vi "SVG Editing Playground.vi"() -> ()   [LabVIEW 2019]
uses:
  Classes/Parse/Image/SVGImage.lvclass
  Classes/Parse/ParseXML/ParseSVG.lvclass
  Classes/Parse/ParseXML/Image.ctl
  <vilib>/LabVIEW Open Source Project/Unicity/UniqueName/UniqueNameClass/Key.ctl
  <vilib>/LabVIEW Open Source Project/Unicity/UniqueName/UniquenessCriteria/Criteria.ctl
  Classes/Parse/ParseXML/ParseSVG.lvclass/ParseSVG.ctl
  <vilib>/LabVIEW Open Source Project/Unicity/UniqueName/UniqueNameClass/UniqueName.lvclass/UniqueName.ctl
  Classes/Parse/Image/InitializationInfo.ctl
  Classes/Parse/EditSVG/EditSVG.lvclass
  <vilib>/LabVIEW Open Source Project/Unicity/UniqueName/Registry/NameRegistry.lvclass
  <vilib>/LabVIEW Open Source Project/Unicity/UniqueName/UniqueNameClass/UniqueName.lvclass
  <vilib>/LabVIEW Open Source Project/Unicity/UniqueName/UniquenessCriteria/UniquenessCriteria.lvclass
panel:
  out "after substring":string
  out "offset past match 5":i32
  out "offset past match 4":i32
  out "offset past match 3":i32
  out "offset past match 2":i32
  out "Array 4":string[](array[string])
  out "Array 3":i32[](array[numeric])
  out "Array 2":i32[](array[numeric])
  out "Array":i32[](array[numeric])
  out "offset past match":i32
  out "Groups":T1(array[cluster])
  out "Path End":i32[](array[numeric])
  out "path start":i32[](array[numeric])
  in  "RawXML":string
  out "Edited in":string
  out "Background Image":refnum<class "SVGImage.lvclass">
  out "error out":errorcluster
  # "ff d8 ff e0 00 10 4a 46 49 46 00 01 01 00 00 01 00 01 00 00 ff fe 00 2d"
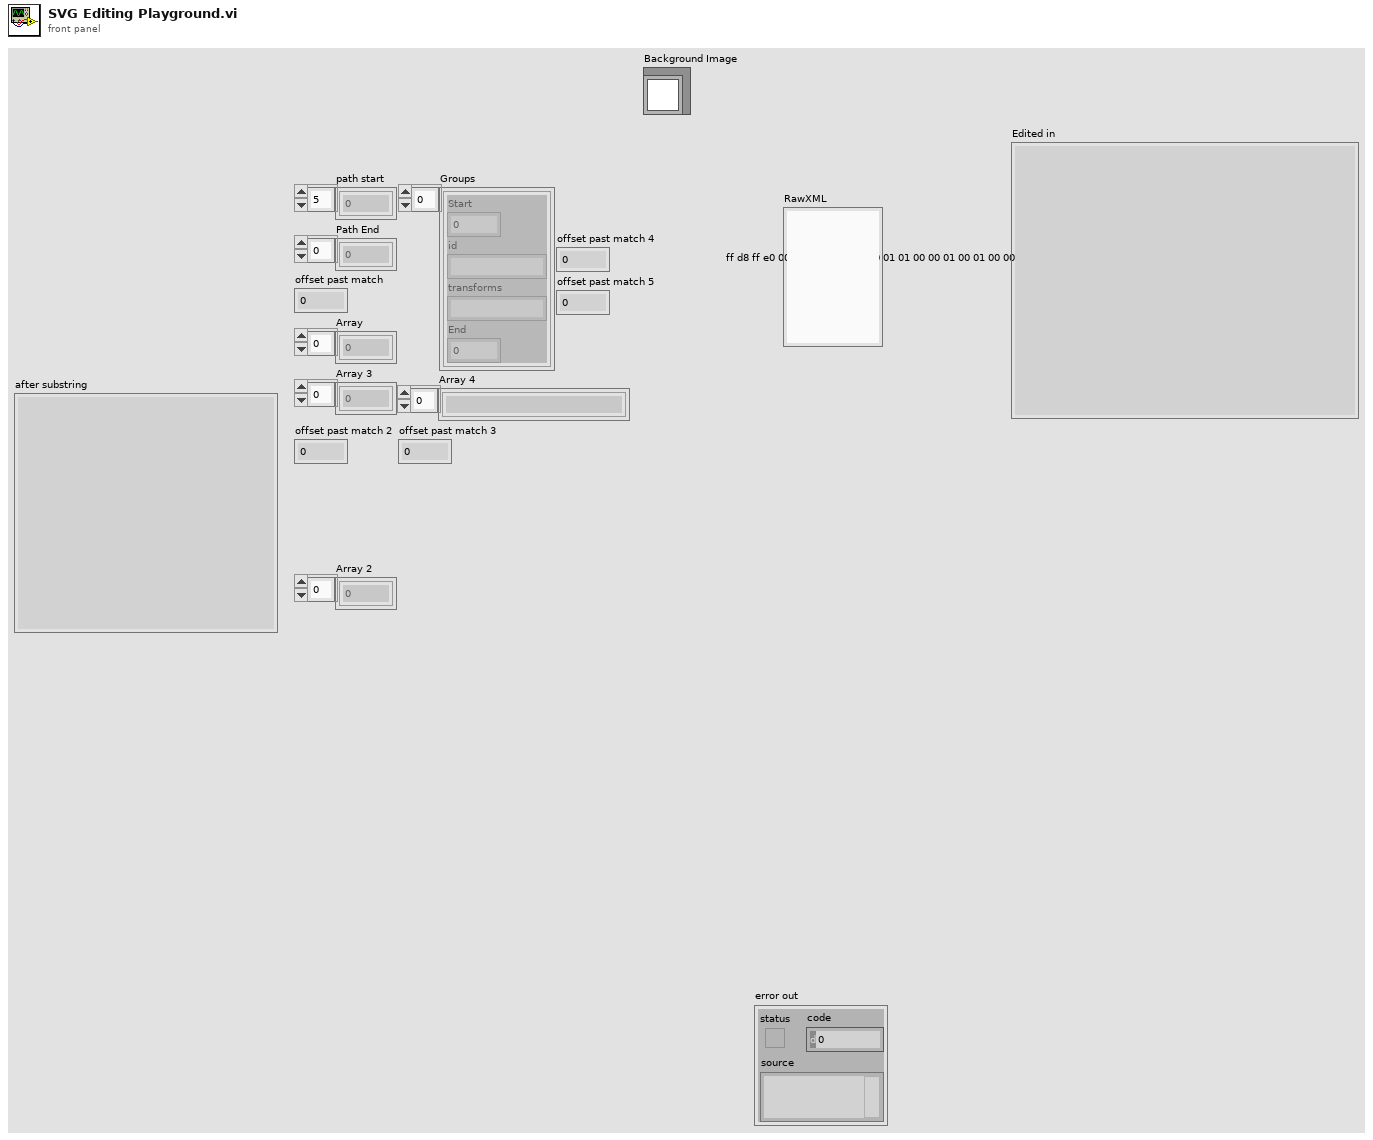
[diagram p1: front panel]
types:
  T1 = cluster{"Start":i32, "id":string, "transforms":string, "End":i32}[]
  T2 = typedef "UniqueName.lvlib/UniquenessCriteria.lvclass/Criteria.ctl" = enum16{"Globally-Unique Fully Qualified Name", "Globally-Unique Name", "Universal Unique Identifier"}
  T3 = typedef "UniqueName.lvlib/UniqueName.lvclass/Key.ctl" = enum16{"Fully Qualified Name", "Unique Name", "Given Name", "Parent Fully Qualified Name", "UUID"}
  T4 = cluster{"Start":i32, "attributes":string, "End":i32}
  T5 = typedef "ParseSVG.lvclass/Image.ctl" = cluster{"x":string, "y":string, "width":string, "height":string, "xlink:href":string, "id":string, "transform":string}
  T6 = typedef "UniqueName.lvlib/NameRegistry.lvclass/RegistryConfiguration.ctl" = cluster{"Delimiter":refnum<class "Delimiter.lvclass">, "RandomStringGenerator":refnum<class "RandomStringGenerator.lvclass">, "UniquenessCriteria":refnum<class "UniquenessCriteria.lvclass">, "StringIncrement":refnum<class "StringIncrement.lvclass">}
  T7 = typedef "SVGImage.lvclass/InitializationInfo.ctl" = cluster{"X":string, "Y":string, "Width":string, "Height":string, "File Path":string, "ID":string, "transform":string}
  T8 = cluster{"Backmost?":bool, "Correct location?":bool, "Surface Pic?":bool, "Correct Name?":bool}
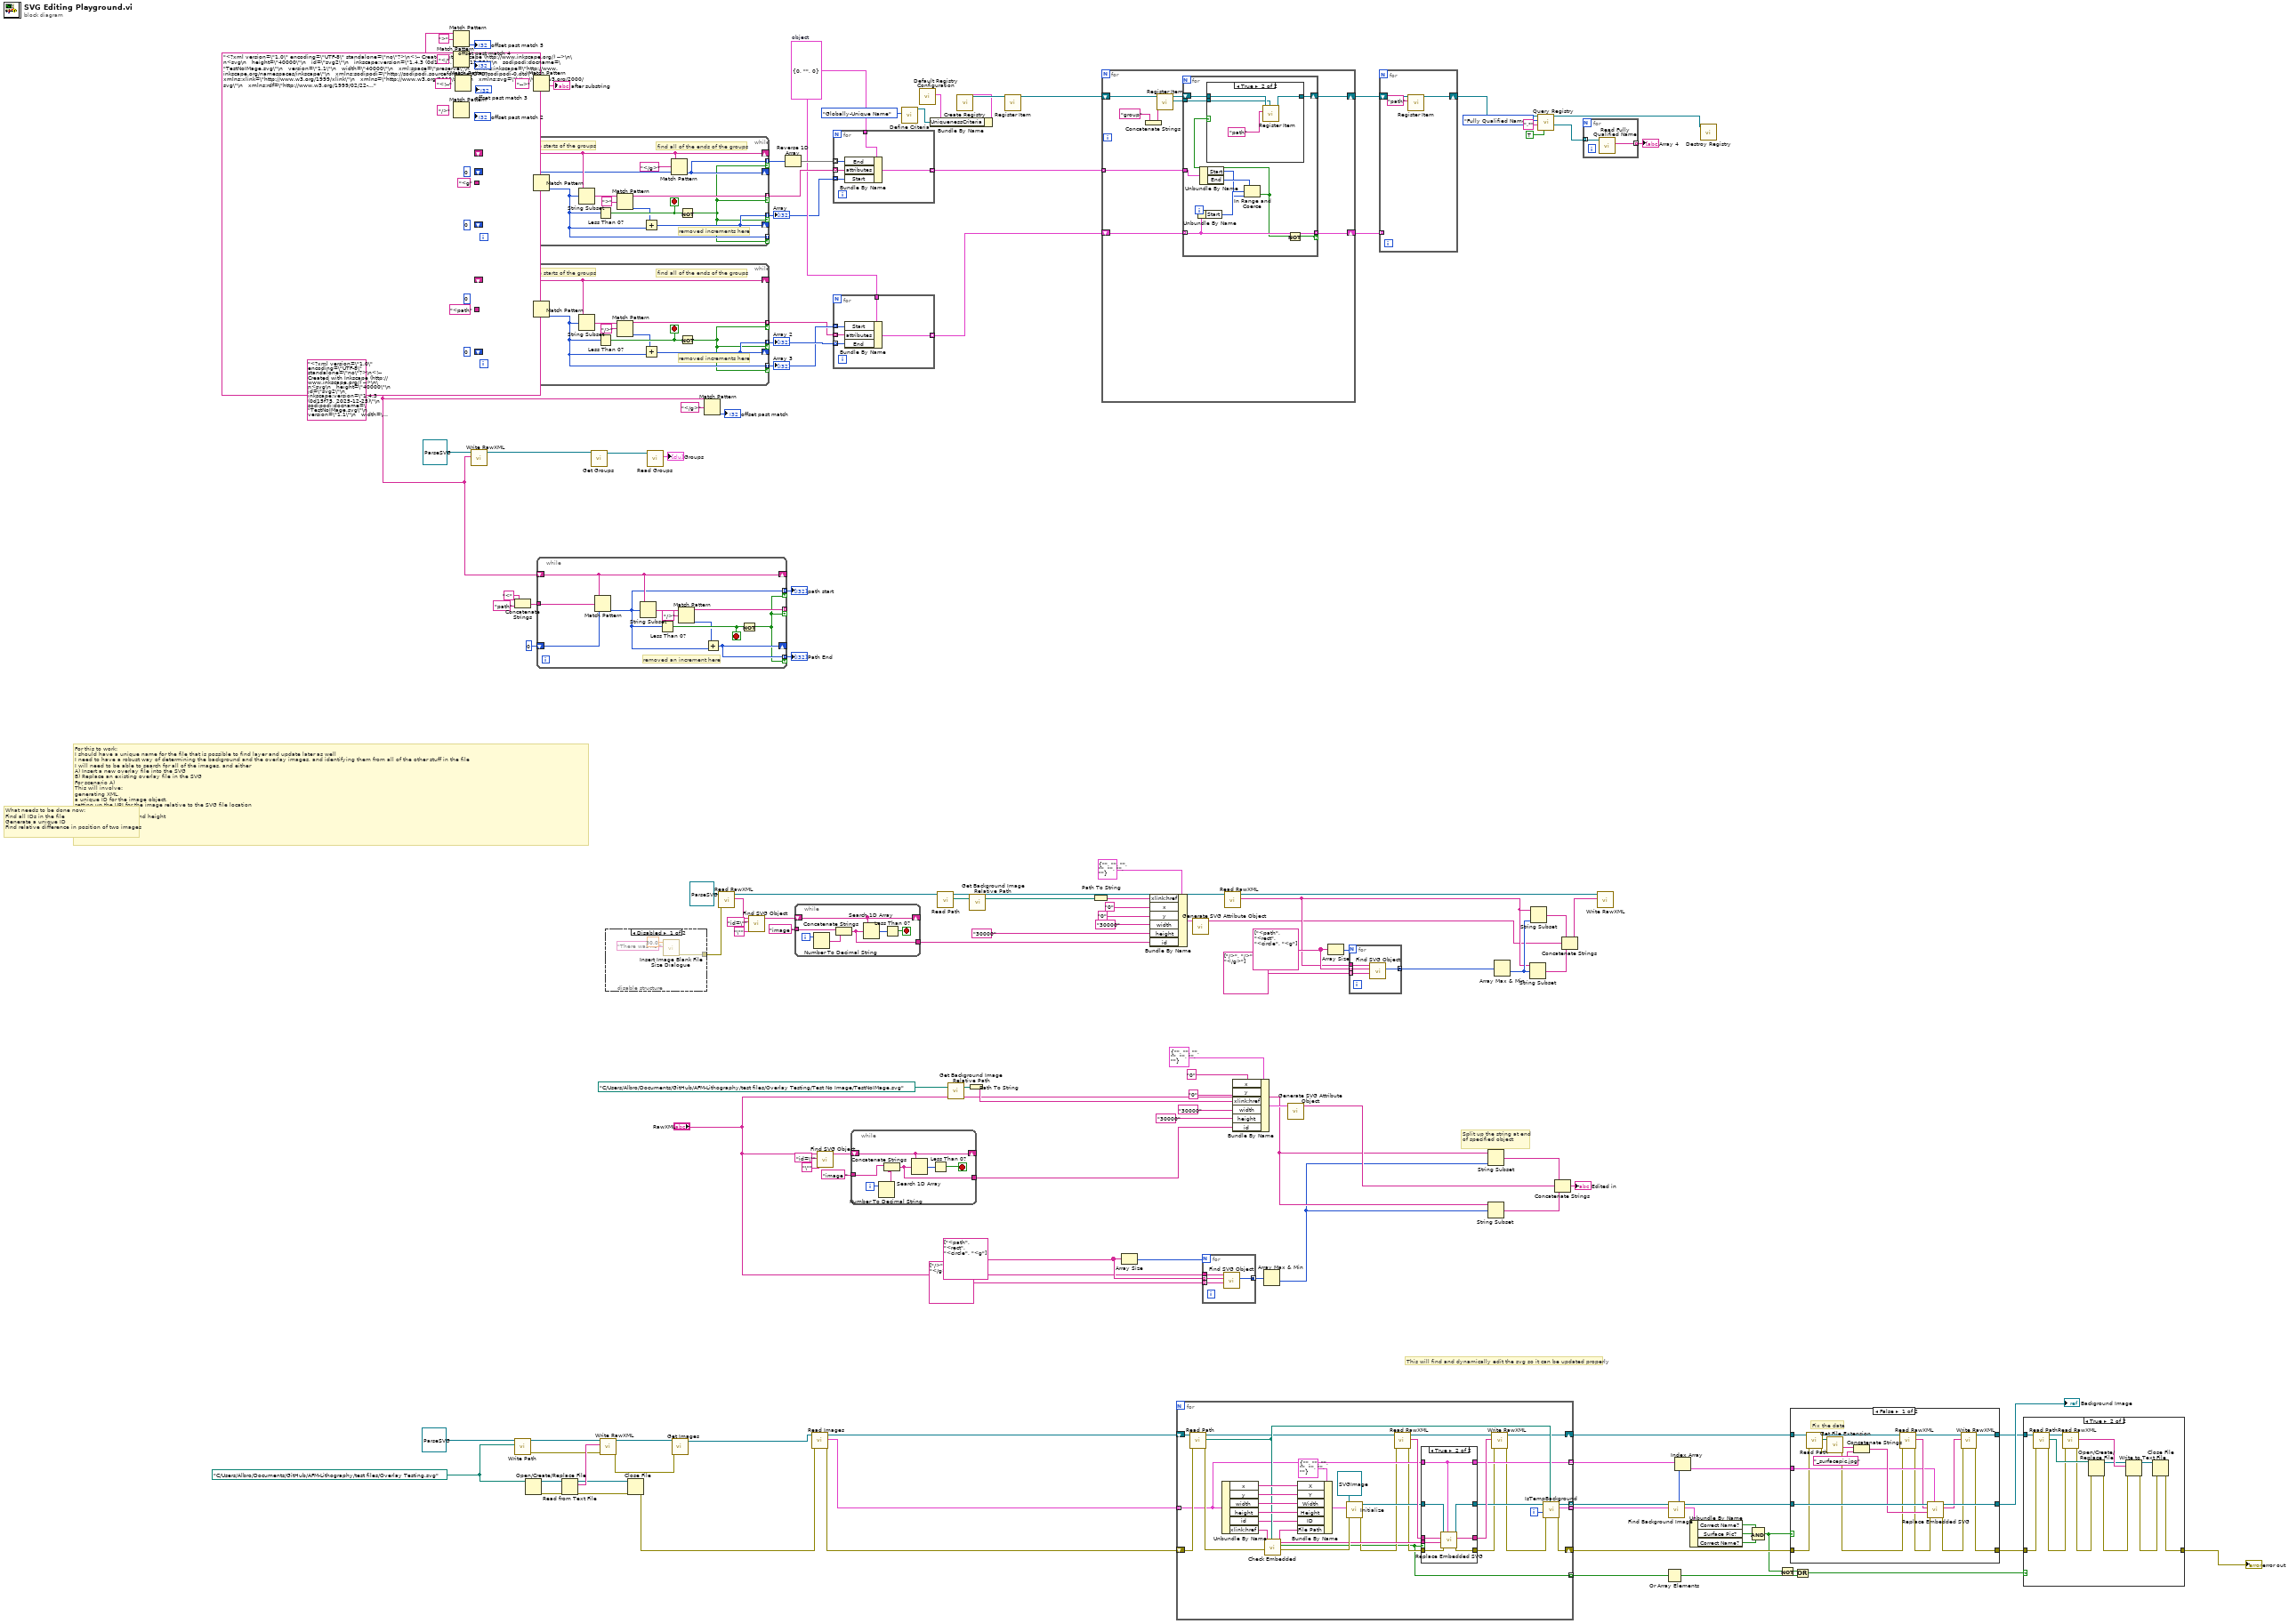
[diagram p0: block diagram]
diagram:
  w8 = "<?xml version=\"1.0\" encoding=\"UTF-8\" standalone=\"no\"?>\n<!-- Created with Inkscape (http://www.inkscape.org/) -->\n\n<svg\n   height=\"40000\"\n   id=\"svg2\"\n   inkscape:version=\"1.4.3 (0d15f75, 2025-12-25)\"\n   sodipodi:docname=\"TestNoIMage.svg\"\n   version=\"1.1\"\n   width=\"40000\"\n   xml:space=\"preserve\"\n   xmlns:inkscape=\"http://www.inkscape.org/namespaces/inkscape\"\n   xmlns:sodipodi=\"http://sodipodi.sourceforge.net/DTD/sodipodi-0.dtd\"\n   xmlns:xlink=\"http://www.w3.org/1999/xlink\"\n   xmlns=\"http://www.w3.org/2000/svg\"\n   xmlns:svg=\"http://www.w3.org/2000/svg\"\n   xmlns:rdf=\"http://www.w3.org/1999/02/22-rdf-syntax-ns#\"\n   xmlns:cc=\"http://creativecommons.org/ns#\"\n   xmlns:dc=\"http://purl.org/dc/elements/1.1/\"><sodipodi:namedview\n     bordercolor=\"#666666\"\n     borderopacity=\"1.0\"\n     id=\"base\"\n     inkscape:current-layer=\"svg2\"\n     inkscape:cx=\"5250\"\n     inkscape:cy=\"13700\"\n     inkscape:deskcolor=\"#d1d1d1\"\n     inkscape:document-units=\"px\"\n     inkscape:pagecheckerboard=\"0\"\n     inkscape:pageopacity=\"0.0\"\n     inkscape:pageshadow=\"2\"\n     inkscape:showpageshadow=\"false\"\n     inkscape:window-height=\"991\"\n     inkscape:window-maximized=\"1\"\n     inkscape:window-width=\"1920\"\n     inkscape:window-x=\"-9\"\n     inkscape:window-y=\"-9\"\n     inkscape:zoom=\"0.01\"\n     pagecolor=\"#ffffff\"\n     showgrid=\"false\" /><defs\n     id=\"defs4\" /><metadata\n     id=\"metadata7\"><rdf:RDF><cc:Work\n         rdf:about=\"\"><dc:format>image/svg+xml</dc:format><dc:type\n           rdf:resource=\"http://purl.org/dc/dcmitype/StillImage\" /></cc:Work></rdf:RDF></metadata><image\n     x=\"0\"\n     y=\"0\"\n     width=\"40000\"\n     height=\"40000\"\n     xlink:href=\"TestNoIMage_surfacepic.jpg\"\n     id=\"image 0\" /><path\n     d=\"m 5710.9429,17975.706 44.593,-4593.756 c 1461.0246,971.983 3035.6976,1713.83 4682.3101,2310.003 -1752.8115,344.069 -3431.5235,862.613 -4726.9031,2283.753 z\"\n     id=\"path3768\"\n     inkscape:connector-curvature=\"0\"\n     sodipodi:nodetypes=\"cccc\"\n     style=\"fill:#00ff00;fill-opacity:1;stroke:#00fb00;stroke-width:68.42746735;stroke-linecap:butt;stroke-linejoin:miter;stroke-miterlimit:4;stroke-dasharray:none;stroke-opacity:1\" /><path\n     d=\"m 13400.892,10059.383 4593.756,44.594 c -971.983,1461.024 -1713.83,3035.698 -2310.003,4682.311 -344.069,-1752.812 -862.613,-3431.524 -2283.753,-4726.905 z\"\n     id=\"path3768-1\"\n     inkscape:connector-curvature=\"0\"\n     sodipodi:nodetypes=\"cccc\"\n     style=\"fill:#00ff00;fill-opacity:1;stroke:#00fb00;stroke-width:68.42746735;stroke-linecap:butt;stroke-linejoin:miter;stroke-miterlimit:4;stroke-dasharray:none;stroke-opacity:1\" /><path\n     d=\"m 18739.549,9988.6728 4593.756,44.5932 c -971.983,1461.025 -1713.83,3035.698 -2310.003,4682.311 -344.069,-1752.812 -862.613,-3431.524 -2283.753,-4726.9042 z\"\n     id=\"path3768-9\"\n     inkscape:connector-curvature=\"0\"\n     sodipodi:nodetypes=\"cccc\"\n     style=\"fill:#00ff00;fill-opacity:1;stroke:#00fb00;stroke-width:68.42746735;stroke-linecap:butt;stroke-linejoin:miter;stroke-miterlimit:4;stroke-dasharray:none;stroke-opacity:1\" /><path\n     d=\"m 8100.4383,10879.12 4509.0037,-879.4745 c -658.548,1626.5485 -1068.815,3318.1785 -1321.924,5051.0065 -689.294,-1647.91 -1534.6121,-3188.17 -3187.0797,-4171.532 z\"\n     id=\"path3768-88\"\n     inkscape:connector-curvature=\"0\"\n     sodipodi:nodetypes=\"cccc\"\n     style=\"fill:#00ff00;fill-opacity:1;stroke:#00fb00;stroke-width:68.42746735;stroke-linecap:butt;stroke-linejoin:miter;stroke-miterlimit:4;stroke-dasharray:none;stroke-opacity:1\" /><path\n     d=\"M 28994.557,10486.846 25071.601,9220.3251 c 541.997,1669.0069 177.663,3332.3599 307.727,5078.7399 803.986,-1595.099 1897.423,-2948.05 3615.229,-3812.219 z\"\n     id=\"path3768-88-4\"\n     inkscape:connector-curvature=\"0\"\n     sodipodi:nodetypes=\"cccc\"\n     style=\"fill:#00ff00;fill-opacity:1;stroke:#00fb00;stroke-width:68.4275;stroke-linecap:butt;stroke-linejoin:miter;stroke-miterlimit:4;stroke-dasharray:none;stroke-opacity:1\" /><path\n     d=\"m 31708.383,17654.207 -44.593,-4593.756 c -1461.024,971.983 -3035.697,1713.83 -4682.31,2310.003 1752.812,344.069 3431.524,862.613 4726.903,2283.753 z\"\n     id=\"path3768-3\"\n     inkscape:connector-curvature=\"0\"\n     sodipodi:nodetypes=\"cccc\"\n     style=\"fill:#00ff00;fill-opacity:1;stroke:#00fb00;stroke-width:68.42746735;stroke-linecap:butt;stroke-linejoin:miter;stroke-miterlimit:4;stroke-dasharray:none;stroke-opacity:1\" /><path\n     d=\"m 9075.4469,21348.552 c 0,0 -5.0869,-1278.12 199.2302,-1901.329 280.3951,-855.263 106.6737,-1996.952 1394.6099,-2478.519 1377.731,-515.142 5080.057,-279.059 7627.666,-339.523 1876.994,-44.548 3759.094,-71.272 5635.365,-16.976 1209.741,35.007 2679.222,-238.229 3614.603,220.69 903.916,443.482 984.374,1305.486 1024.612,2003.186 44.859,777.835 -882.304,2274.805 -882.304,2274.805\"\n     id=\"path3856\"\n     inkscape:connector-curvature=\"0\"\n     sodipodi:nodetypes=\"casaaaac\"\n     style=\"fill:none;stroke:#00fb00;stroke-width:62.17174911;stroke-linecap:butt;stroke-linejoin:miter;stroke-miterlimit:4;stroke-dasharray:none;stroke-opacity:1\" /><rect\n     height=\"7255.8125\"\n     id=\"rect14\"\n     style=\"opacity:1;fill:#00ff00;fill-opacity:1;stroke:#000000;stroke-width:0.755906;stroke-miterlimit:4;stroke-dasharray:none;stroke-opacity:1\"\n     width=\"11888.403\"\n     x=\"14347.161\"\n     y=\"20973.98\" /><rect\n     height=\"7253.042\"\n     id=\"rect14-8\"\n     style=\"fill:#00ff00;fill-opacity:1;stroke:#000000;stroke-width:0.693561;stroke-miterlimit:4;stroke-dasharray:none;stroke-opacity:1\"\n     transform=\"matrix(1.1237265,-0.00330692,0.45761161,1.2541239,-10097.789,-20728.359)\"\n     width=\"10291.699\"\n     x=\"-4974.5957\"\n     y=\"39154.031\" /><text\n     id=\"text843\"\n     style=\"font-style:normal;font-weight:normal;font-size:53.3333px;line-height:1.25;font-family:sans-serif;letter-spacing:0px;word-spacing:0px;fill:#000000;fill-opacity:1;stroke:none\"\n     x=\"12020.815\"\n     xml:space=\"preserve\"\n     y=\"20554.562\">\n    <tspan\n   id=\"tspan841\"\n   sodipodi:role=\"line\"\n   x=\"12020.815\"\n   y=\"20554.562\">T</tspan>\n  </text><circle\n     cx=\"15000\"\n     cy=\"18500\"\n     id=\"path825\"\n     r=\"100\"\n     style=\"opacity:1;fill:#00ff00;fill-opacity:1;stroke:#000000;stroke-width:1.00157;stroke-miterlimit:4;stroke-dasharray:none;stroke-opacity:1\" /><circle\n     cx=\"20000\"\n     cy=\"18500\"\n     id=\"path825-31\"\n     r=\"100\"\n     style=\"fill:#00ff00;fill-opacity:1;stroke:#000000;stroke-width:1.00157;stroke-miterlimit:4;stroke-dasharray:none;stroke-opacity:1\" /><circle\n     cx=\"22500\"\n     cy=\"18500\"\n     id=\"path825-3\"\n     r=\"100\"\n     style=\"fill:#00ff00;fill-opacity:1;stroke:#000000;stroke-width:1.00157;stroke-miterlimit:4;stroke-dasharray:none;stroke-opacity:1\" /><circle\n     cx=\"17500\"\n     cy=\"18500\"\n     id=\"path825-9\"\n     r=\"100\"\n     style=\"fill:#00ff00;fill-opacity:1;stroke:#000000;stroke-width:1.00157;stroke-miterlimit:4;stroke-dasharray:none;stroke-opacity:1\" /><circle\n     cx=\"25000\"\n     cy=\"18500\"\n     id=\"path825-3-5\"\n     r=\"100\"\n     style=\"fill:#00ff00;fill-opacity:1;stroke:#000000;stroke-width:1.00157;stroke-miterlimit:4;stroke-dasharray:none;stroke-opacity:1\" /><circle\n     cx=\"13000\"\n     cy=\"20500\"\n     id=\"path825-5\"\n     r=\"100\"\n     style=\"fill:#00ff00;fill-opacity:1;stroke:#000000;stroke-width:1.00157;stroke-miterlimit:4;stroke-dasharray:none;stroke-opacity:1\" /><circle\n     cx=\"17000\"\n     cy=\"20500\"\n     id=\"path825-3-4\"\n     r=\"100\"\n     style=\"fill:#00ff00;fill-opacity:1;stroke:#000000;stroke-width:1.00157;stroke-miterlimit:4;stroke-dasharray:none;stroke-opacity:1\" /><circle\n     cx=\"15000\"\n     cy=\"20500\"\n     id=\"path825-9-6\"\n     r=\"100\"\n     style=\"fill:#00ff00;fill-opacity:1;stroke:#000000;stroke-width:1.00157;stroke-miterlimit:4;stroke-dasharray:none;stroke-opacity:1\" /><circle\n     cx=\"19000\"\n     cy=\"20500\"\n     id=\"path825-3-5-2\"\n     r=\"100\"\n     style=\"fill:#00ff00;fill-opacity:1;stroke:#000000;stroke-width:1.00157;stroke-miterlimit:4;stroke-dasharray:none;stroke-opacity:1\" /><path\n     d=\"M 13650,17000 26000,15600\"\n     id=\"path1392\"\n     inkscape:connector-curvature=\"0\"\n     style=\"fill:none;stroke:#00ff00;stroke-width:50;stroke-linecap:butt;stroke-linejoin:miter;stroke-miterlimit:4;stroke-dasharray:none;stroke-opacity:1\" /><path\n     d=\"m 11200,26850 c 1203.007,3334.458 2168.666,2633.989 3250,3900 l 3300,-1750\"\n     id=\"path1394\"\n     inkscape:connector-curvature=\"0\"\n     sodipodi:nodetypes=\"ccc\"\n     style=\"fill:none;stroke:#00ff00;stroke-width:50;stroke-linecap:butt;stroke-linejoin:miter;stroke-miterlimit:4;stroke-dasharray:none;stroke-opacity:1\" /><path\n     d=\"m 14849.242,3959.7979 h 11525.84\"\n     id=\"path4\"\n     style=\"fill:none;stroke:#00ff00;stroke-width:100px;stroke-linecap:butt;stroke-linejoin:miter;stroke-opacity:1\"\n     transform=\"translate(0,440)\" /><path\n     d=\"M 14849.242,4560.8386 H 26357.405\"\n     id=\"path2\"\n     style=\"fill:none;stroke:#00FF00;stroke-width:100px;stroke-linecap:butt;stroke-linejoin:miter;stroke-opacity:1\" /><g\n     id=\"g1\"\n     transform=\"matrix(0.97420092,0,0,1.1904169,383.55282,-892.60137)\"><path\n       d=\"M 14850,5174.9999 H 26349.999\"\n       id=\"path1\"\n       style=\"fill:none;stroke:#00ff00;stroke-width:100px;stroke-linecap:butt;stroke-linejoin:miter;stroke-opacity:1\"\n       transform=\"translate(16.91967,-437.3846)\" /><g\n       id=\"g3\"\n       transform=\"matrix(0.87240932,-0.1215228,0.11425413,0.92791062,3276.3322,3478.6107)\"><path\n         d=\"m 14849.242,3959.7979 h 11525.84\"\n         id=\"path4-6\"\n         style=\"fill:none;stroke:#00ff00;stroke-width:100px;stroke-linecap:butt;stroke-linejoin:miter;stroke-opacity:1\"\n         transform=\"translate(4993.758,1820.2021)\" /><path\n         d=\"M 14849.242,4560.8386 H 26357.405\"\n         id=\"path2-3\"\n         style=\"fill:none;stroke:#00ff00;stroke-width:100px;stroke-linecap:butt;stroke-linejoin:miter;stroke-opacity:1\"\n         transform=\"translate(4993.758,1380.2021)\" /><path\n         d=\"M 14850,5174.9999 H 26349.999\"\n         id=\"path1-6\"\n         style=\"fill:none;stroke:#00ff00;stroke-width:100px;stroke-linecap:butt;stroke-linejoin:miter;stroke-opacity:1\"\n         transform=\"translate(5010.6777,942.8175)\" /></g></g><path\n     d=\"M 19657.6 32703.7 C 19692.2 32408.2 19726.9 32124.8 19761.6 32036.9 C 19796.2 31949 19830.9 32064.5 19865.6 32307.7 C 19900.2 32551 19934.9 32903 19969.6 33135.3 C 20004.2 33367.7 20038.9 33461.2 20073.6 33356 C 20108.2 33250.7 20142.9 32954.3 20177.6 32659.4 C 20212.2 32364.5 20246.9 32094.9 20281.6 32025.1 C 20316.2 31955.3 20350.9 32091.6 20385.6 32345 C 20420.2 32598.4 20454.9 32949 20489.6 33169.3 C 20524.3 33389.6 20558.9 33461.4 20593.6 33338.9 C 20628.3 33216.3 20662.9 32908.4 20697.6 32615.3 C 20732.3 32322.2 20766.9 32067.5 20801.6 32016 C 20836.3 31964.5 20870.9 32121.2 20905.6 32383.7 C 20940.3 32646.2 20974.9 32994 21009.6 33201.3 C 21044.3 33408.7 21078.9 33458.5 21113.6 33319.2 C 21148.3 33179.8 21182.9 32861.7 21217.6 32571.5 C 21252.3 32281.4 21286.9 32042.7 21321.6 32009.7 C 21356.3 31976.8 21390.9 32153.1 21425.6 32423.7 C 21460.3 32694.3 21494.9 33037.8 21529.6 33231.4 C 21564.3 33425 21598.9 33452.6 21633.6 33297 C 21668.3 33141.4 21702.9 32814.3 21737.6 32528.3 C 21772.3 32242.3 21806.9 32020.5 21841.6 32006.2 C 21876.3 31992 21910.9 32187.3 21945.6 32464.9 C 21980.3 32742.4 22014.9 33080.3 22049.6 33259.3 C 22084.3 33438.4 22119 33443.7 22153.6 33272.5 C 22188.3 33101.3 22223 32766.6 22257.6 32485.8 C 22292.3 32205.1 22327 32001 22361.6 32005.5 C 22396.3 32010 22431 32223.5 22465.6 32507 C 22500.3 32790.4 22535 33121.2 22569.6 33285 C 22604.3 33448.9 22639 33431.8 22673.6 33245.6 C 22708.3 33059.5 22743 32718.5 22777.6 32444.2 C 22812.3 32169.8 22847 31984.4 22881.6 32007.6 C 22916.3 32030.8 22951 32261.7 22985.6 32549.9 C 23020.3 32838 23055 33160.5 23089.6 33308.4 C 23124.3 33456.3 23159 33417 23193.6 33216.6 C 23228.3 33016.3 23263 32670.4 23297.6 32403.6 C 23332.3 32136.7 23367 31970.7 23401.6 32012.5 C 23436.3 32054.4 23471 32301.7 23505.6 32593.4 C 23540.3 32885.1 23575 33198 23609.6 33329.3 C 23644.3 33460.7 23679 33399.2 23713.6 33185.5 C 23748.3 32971.9 23783 32622.5 23817.7 32364.2 C 23852.3 32105.9 23887 31959.9 23921.7 32020.2 C 23956.3 32080.5 23991 32343.2 24025.7 32637.3 C 24060.3 32931.4 24095 33233.4 24129.7 33347.7 C 24164.3 33462.1 24199 33378.7 24233.7 33152.5 C 24268.3 32926.3 24303 32574.8 24337.7 32326.2 C 24372.3 32077.5 24407 31952.1 24441.7 32030.7 C 24476.3 32109.2 24511 32386.2 24545.7 32681.5 C 24580.3 32976.8 24615 33266.7 24649.7 33363.6 C 24684.3 33460.4 24719 33355.5 24753.7 33117.7 C 24788.3 32879.9 24823 32527.7 24857.7 32289.7 C 24892.3 32051.7 24927 31947.4 24961.7 32043.8 C 24996.3 32140.3 25031 32430.5 25065.7 32725.8 C 25100.3 33021.1 25135 33297.8 25169.7 33376.7 C 25204.3 33455.6 25239 33329.6 25273.7 33081.2 C 25308.3 32832.8 25343 32481.3 25377.7 32254.9 C 25412.3 32028.4 25447 31945.7 25481.7 32059.6 C 25516.4 32173.6 25551 32475.9 25585.7 32770.1 C 25620.4 33064.2 25655 33326.5 25689.7 33387.2 C 25724.4 33447.8 25759 33301.3 25793.7 33043.2 C 25828.4 32785.1 25863 32435.8 25897.7 32221.8 C 25932.4 32007.9 25967 31947 26001.7 32078 C 26036.4 32209.1 26071 32522.3 26105.7 32814 C 26140.4 33105.8 26175 33352.6 26209.7 33394.8 C 26244.4 33437.1 26279 33270.5 26313.7 33003.8 C 26348.4 32737.1 26383 32391.3 26417.7 32190.7 C 26452.4 31990.1 26487 31951.4 26521.7 32099 C 26556.4 32246.5 26591 32569.3 26625.7 32857.5 C 26660.4 33145.8 26695 33376.2 26729.7 33399.8 C 26764.4 33423.4 26799 33237.4 26833.7 32963.2 C 26868.4 32689 26903 32348.2 26937.7 32161.7 C 26972.4 31975.3 27007 31958.8 27041.7 32122.3 C 27076.4 32285.8 27111 32616.9 27145.7 32900.4 C 27180.4 33183.9 27215.1 33397 27249.7 33401.9 C 27284.4 33406.7 27319.1 33202.2 27353.7 32921.6 C 27388.4 32640.9 27423.1 32306.4 27457.7 32134.9 C 27492.4 31963.4 27527.1 31969.3 27561.7 32148 C 27596.4 32326.8 27631.1 32664.8 27665.7 32942.5 C 27700.4 33220.2 27735.1 33415 27769.7 33401.2 C 27804.4 33387.3 27839.1 33165 27873.7 32879.1 C 27908.4 32593.1 27943.1 32266.3 27977.7 32110.4 C 28012.4 31954.4 28047.1 31982.6 28081.7 32176 C 28116.4 32369.3 28151.1 32712.9 28185.7 32983.6 C 28220.4 33254.4 28255.1 33430.2 28289.7 33397.7 C 28324.4 33365.1 28359.1 33125.9 28393.7 32835.8 C 28428.4 32545.8 28463.1 32227.9 28497.7 32088.2 C 28532.4 31948.5 28567.1 31998.9 28601.7 32206 C 28636.4 32413.2 28671.1 32761 28705.7 33023.7 C 28740.4 33286.3 28775.1 33442.5 28809.8 33391.3 C 28844.4 33340.2 28879.1 33085.1 28913.8 32792.1 C 28948.4 32499 28983.1 32191.4 29017.8 32068.5 C 29052.4 31945.6 29087.1 32018 29121.8 32238.1 C 29156.4 32458.2 29191.1 32808.8 29225.8 33062.4 C 29260.4 33316 29295.1 33451.7 29329.8 33382.3 C 29364.4 33312.8 29399.1 33042.8 29433.8 32748 C 29468.4 32453.1 29503.1 32157 29537.8 32051.4 C 29572.4 31945.8 29607.1 32039.9 29641.8 32272 C 29676.4 32504.2 29711.1 32856.2 29745.8 33099.6 C 29780.4 33343.1 29815.1 33458 29849.8 33370.5 C 29884.4 33282.9 29919.1 32999.1 29953.8 32703.7\"\n     id=\"path3\"\n     style=\"fill:none;stroke:#00ff00;stroke-width:100;paint-order:fill markers stroke;stroke-dasharray:none\"\n     title=\"t sin(20*t)\" /></svg>"
  (unwired) 0 ("offset past match")
  w34 = T4 {"Start"=0, "attributes"="", "End"=0}  # object
  w37 = "<?xml version=\"1.0\" encoding=\"UTF-8\" standalone=\"no\"?>\n<!-- Created with Inkscape (http://www.inkscape.org/) -->\n\n<svg\n   height=\"40000\"\n   id=\"svg2\"\n   inkscape:version=\"1.4.3 (0d15f75, 2025-12-25)\"\n   sodipodi:docname=\"TestNoIMage.svg\"\n   version=\"1.1\"\n   width=\"40000\"\n   xml:space=\"preserve\"\n   xmlns:inkscape=\"http://www.inkscape.org/namespaces/inkscape\"\n   xmlns:sodipodi=\"http://sodipodi.sourceforge.net/DTD/sodipodi-0.dtd\"\n   xmlns:xlink=\"http://www.w3.org/1999/xlink\"\n   xmlns=\"http://www.w3.org/2000/svg\"\n   xmlns:svg=\"http://www.w3.org/2000/svg\"\n   xmlns:rdf=\"http://www.w3.org/1999/02/22-rdf-syntax-ns#\"\n   xmlns:cc=\"http://creativecommons.org/ns#\"\n   xmlns:dc=\"http://purl.org/dc/elements/1.1/\"><sodipodi:namedview\n     bordercolor=\"#666666\"\n     borderopacity=\"1.0\"\n     id=\"base\"\n     inkscape:current-layer=\"svg2\"\n     inkscape:cx=\"5250\"\n     inkscape:cy=\"13700\"\n     inkscape:deskcolor=\"#d1d1d1\"\n     inkscape:document-units=\"px\"\n     inkscape:pagecheckerboard=\"0\"\n     inkscape:pageopacity=\"0.0\"\n     inkscape:pageshadow=\"2\"\n     inkscape:showpageshadow=\"false\"\n     inkscape:window-height=\"991\"\n     inkscape:window-maximized=\"1\"\n     inkscape:window-width=\"1920\"\n     inkscape:window-x=\"-9\"\n     inkscape:window-y=\"-9\"\n     inkscape:zoom=\"0.01\"\n     pagecolor=\"#ffffff\"\n     showgrid=\"false\" /><defs\n     id=\"defs4\" /><metadata\n     id=\"metadata7\"><rdf:RDF><cc:Work\n         rdf:about=\"\"><dc:format>image/svg+xml</dc:format><dc:type\n           rdf:resource=\"http://purl.org/dc/dcmitype/StillImage\" /></cc:Work></rdf:RDF></metadata><image\n     x=\"0\"\n     y=\"0\"\n     width=\"40000\"\n     height=\"40000\"\n     xlink:href=\"TestNoIMage_surfacepic.jpg\"\n     id=\"image 0\" /><path\n     d=\"m 5710.9429,17975.706 44.593,-4593.756 c 1461.0246,971.983 3035.6976,1713.83 4682.3101,2310.003 -1752.8115,344.069 -3431.5235,862.613 -4726.9031,2283.753 z\"\n     id=\"path3768\"\n     inkscape:connector-curvature=\"0\"\n     sodipodi:nodetypes=\"cccc\"\n     style=\"fill:#00ff00;fill-opacity:1;stroke:#00fb00;stroke-width:68.42746735;stroke-linecap:butt;stroke-linejoin:miter;stroke-miterlimit:4;stroke-dasharray:none;stroke-opacity:1\" /><path\n     d=\"m 13400.892,10059.383 4593.756,44.594 c -971.983,1461.024 -1713.83,3035.698 -2310.003,4682.311 -344.069,-1752.812 -862.613,-3431.524 -2283.753,-4726.905 z\"\n     id=\"path3768-1\"\n     inkscape:connector-curvature=\"0\"\n     sodipodi:nodetypes=\"cccc\"\n     style=\"fill:#00ff00;fill-opacity:1;stroke:#00fb00;stroke-width:68.42746735;stroke-linecap:butt;stroke-linejoin:miter;stroke-miterlimit:4;stroke-dasharray:none;stroke-opacity:1\" /><path\n     d=\"m 18739.549,9988.6728 4593.756,44.5932 c -971.983,1461.025 -1713.83,3035.698 -2310.003,4682.311 -344.069,-1752.812 -862.613,-3431.524 -2283.753,-4726.9042 z\"\n     id=\"path3768-9\"\n     inkscape:connector-curvature=\"0\"\n     sodipodi:nodetypes=\"cccc\"\n     style=\"fill:#00ff00;fill-opacity:1;stroke:#00fb00;stroke-width:68.42746735;stroke-linecap:butt;stroke-linejoin:miter;stroke-miterlimit:4;stroke-dasharray:none;stroke-opacity:1\" /><path\n     d=\"m 8100.4383,10879.12 4509.0037,-879.4745 c -658.548,1626.5485 -1068.815,3318.1785 -1321.924,5051.0065 -689.294,-1647.91 -1534.6121,-3188.17 -3187.0797,-4171.532 z\"\n     id=\"path3768-88\"\n     inkscape:connector-curvature=\"0\"\n     sodipodi:nodetypes=\"cccc\"\n     style=\"fill:#00ff00;fill-opacity:1;stroke:#00fb00;stroke-width:68.42746735;stroke-linecap:butt;stroke-linejoin:miter;stroke-miterlimit:4;stroke-dasharray:none;stroke-opacity:1\" /><path\n     d=\"M 28994.557,10486.846 25071.601,9220.3251 c 541.997,1669.0069 177.663,3332.3599 307.727,5078.7399 803.986,-1595.099 1897.423,-2948.05 3615.229,-3812.219 z\"\n     id=\"path3768-88-4\"\n     inkscape:connector-curvature=\"0\"\n     sodipodi:nodetypes=\"cccc\"\n     style=\"fill:#00ff00;fill-opacity:1;stroke:#00fb00;stroke-width:68.4275;stroke-linecap:butt;stroke-linejoin:miter;stroke-miterlimit:4;stroke-dasharray:none;stroke-opacity:1\" /><path\n     d=\"m 31708.383,17654.207 -44.593,-4593.756 c -1461.024,971.983 -3035.697,1713.83 -4682.31,2310.003 1752.812,344.069 3431.524,862.613 4726.903,2283.753 z\"\n     id=\"path3768-3\"\n     inkscape:connector-curvature=\"0\"\n     sodipodi:nodetypes=\"cccc\"\n     style=\"fill:#00ff00;fill-opacity:1;stroke:#00fb00;stroke-width:68.42746735;stroke-linecap:butt;stroke-linejoin:miter;stroke-miterlimit:4;stroke-dasharray:none;stroke-opacity:1\" /><path\n     d=\"m 9075.4469,21348.552 c 0,0 -5.0869,-1278.12 199.2302,-1901.329 280.3951,-855.263 106.6737,-1996.952 1394.6099,-2478.519 1377.731,-515.142 5080.057,-279.059 7627.666,-339.523 1876.994,-44.548 3759.094,-71.272 5635.365,-16.976 1209.741,35.007 2679.222,-238.229 3614.603,220.69 903.916,443.482 984.374,1305.486 1024.612,2003.186 44.859,777.835 -882.304,2274.805 -882.304,2274.805\"\n     id=\"path3856\"\n     inkscape:connector-curvature=\"0\"\n     sodipodi:nodetypes=\"casaaaac\"\n     style=\"fill:none;stroke:#00fb00;stroke-width:62.17174911;stroke-linecap:butt;stroke-linejoin:miter;stroke-miterlimit:4;stroke-dasharray:none;stroke-opacity:1\" /><rect\n     height=\"7255.8125\"\n     id=\"rect14\"\n     style=\"opacity:1;fill:#00ff00;fill-opacity:1;stroke:#000000;stroke-width:0.755906;stroke-miterlimit:4;stroke-dasharray:none;stroke-opacity:1\"\n     width=\"11888.403\"\n     x=\"14347.161\"\n     y=\"20973.98\" /><rect\n     height=\"7253.042\"\n     id=\"rect14-8\"\n     style=\"fill:#00ff00;fill-opacity:1;stroke:#000000;stroke-width:0.693561;stroke-miterlimit:4;stroke-dasharray:none;stroke-opacity:1\"\n     transform=\"matrix(1.1237265,-0.00330692,0.45761161,1.2541239,-10097.789,-20728.359)\"\n     width=\"10291.699\"\n     x=\"-4974.5957\"\n     y=\"39154.031\" /><text\n     id=\"text843\"\n     style=\"font-style:normal;font-weight:normal;font-size:53.3333px;line-height:1.25;font-family:sans-serif;letter-spacing:0px;word-spacing:0px;fill:#000000;fill-opacity:1;stroke:none\"\n     x=\"12020.815\"\n     xml:space=\"preserve\"\n     y=\"20554.562\">\n    <tspan\n   id=\"tspan841\"\n   sodipodi:role=\"line\"\n   x=\"12020.815\"\n   y=\"20554.562\">T</tspan>\n  </text><circle\n     cx=\"15000\"\n     cy=\"18500\"\n     id=\"path825\"\n     r=\"100\"\n     style=\"opacity:1;fill:#00ff00;fill-opacity:1;stroke:#000000;stroke-width:1.00157;stroke-miterlimit:4;stroke-dasharray:none;stroke-opacity:1\" /><circle\n     cx=\"20000\"\n     cy=\"18500\"\n     id=\"path825-31\"\n     r=\"100\"\n     style=\"fill:#00ff00;fill-opacity:1;stroke:#000000;stroke-width:1.00157;stroke-miterlimit:4;stroke-dasharray:none;stroke-opacity:1\" /><circle\n     cx=\"22500\"\n     cy=\"18500\"\n     id=\"path825-3\"\n     r=\"100\"\n     style=\"fill:#00ff00;fill-opacity:1;stroke:#000000;stroke-width:1.00157;stroke-miterlimit:4;stroke-dasharray:none;stroke-opacity:1\" /><circle\n     cx=\"17500\"\n     cy=\"18500\"\n     id=\"path825-9\"\n     r=\"100\"\n     style=\"fill:#00ff00;fill-opacity:1;stroke:#000000;stroke-width:1.00157;stroke-miterlimit:4;stroke-dasharray:none;stroke-opacity:1\" /><circle\n     cx=\"25000\"\n     cy=\"18500\"\n     id=\"path825-3-5\"\n     r=\"100\"\n     style=\"fill:#00ff00;fill-opacity:1;stroke:#000000;stroke-width:1.00157;stroke-miterlimit:4;stroke-dasharray:none;stroke-opacity:1\" /><circle\n     cx=\"13000\"\n     cy=\"20500\"\n     id=\"path825-5\"\n     r=\"100\"\n     style=\"fill:#00ff00;fill-opacity:1;stroke:#000000;stroke-width:1.00157;stroke-miterlimit:4;stroke-dasharray:none;stroke-opacity:1\" /><circle\n     cx=\"17000\"\n     cy=\"20500\"\n     id=\"path825-3-4\"\n     r=\"100\"\n     style=\"fill:#00ff00;fill-opacity:1;stroke:#000000;stroke-width:1.00157;stroke-miterlimit:4;stroke-dasharray:none;stroke-opacity:1\" /><circle\n     cx=\"15000\"\n     cy=\"20500\"\n     id=\"path825-9-6\"\n     r=\"100\"\n     style=\"fill:#00ff00;fill-opacity:1;stroke:#000000;stroke-width:1.00157;stroke-miterlimit:4;stroke-dasharray:none;stroke-opacity:1\" /><circle\n     cx=\"19000\"\n     cy=\"20500\"\n     id=\"path825-3-5-2\"\n     r=\"100\"\n     style=\"fill:#00ff00;fill-opacity:1;stroke:#000000;stroke-width:1.00157;stroke-miterlimit:4;stroke-dasharray:none;stroke-opacity:1\" /><path\n     d=\"M 13650,17000 26000,15600\"\n     id=\"path1392\"\n     inkscape:connector-curvature=\"0\"\n     style=\"fill:none;stroke:#00ff00;stroke-width:50;stroke-linecap:butt;stroke-linejoin:miter;stroke-miterlimit:4;stroke-dasharray:none;stroke-opacity:1\" /><path\n     d=\"m 11200,26850 c 1203.007,3334.458 2168.666,2633.989 3250,3900 l 3300,-1750\"\n     id=\"path1394\"\n     inkscape:connector-curvature=\"0\"\n     sodipodi:nodetypes=\"ccc\"\n     style=\"fill:none;stroke:#00ff00;stroke-width:50;stroke-linecap:butt;stroke-linejoin:miter;stroke-miterlimit:4;stroke-dasharray:none;stroke-opacity:1\" /><path\n     d=\"m 14849.242,3959.7979 h 11525.84\"\n     id=\"path4\"\n     style=\"fill:none;stroke:#00ff00;stroke-width:100px;stroke-linecap:butt;stroke-linejoin:miter;stroke-opacity:1\"\n     transform=\"translate(0,440)\" /><path\n     d=\"M 14849.242,4560.8386 H 26357.405\"\n     id=\"path2\"\n     style=\"fill:none;stroke:#00FF00;stroke-width:100px;stroke-linecap:butt;stroke-linejoin:miter;stroke-opacity:1\" /><g\n     id=\"g1\"\n     transform=\"matrix(0.97420092,0,0,1.1904169,383.55282,-892.60137)\"><path\n       d=\"M 14850,5174.9999 H 26349.999\"\n       id=\"path1\"\n       style=\"fill:none;stroke:#00ff00;stroke-width:100px;stroke-linecap:butt;stroke-linejoin:miter;stroke-opacity:1\"\n       transform=\"translate(16.91967,-437.3846)\" /><g\n       id=\"g3\"\n       transform=\"matrix(0.87240932,-0.1215228,0.11425413,0.92791062,3276.3322,3478.6107)\"><path\n         d=\"m 14849.242,3959.7979 h 11525.84\"\n         id=\"path4-6\"\n         style=\"fill:none;stroke:#00ff00;stroke-width:100px;stroke-linecap:butt;stroke-linejoin:miter;stroke-opacity:1\"\n         transform=\"translate(4993.758,1820.2021)\" /><path\n         d=\"M 14849.242,4560.8386 H 26357.405\"\n         id=\"path2-3\"\n         style=\"fill:none;stroke:#00ff00;stroke-width:100px;stroke-linecap:butt;stroke-linejoin:miter;stroke-opacity:1\"\n         transform=\"translate(4993.758,1380.2021)\" /><path\n         d=\"M 14850,5174.9999 H 26349.999\"\n         id=\"path1-6\"\n         style=\"fill:none;stroke:#00ff00;stroke-width:100px;stroke-linecap:butt;stroke-linejoin:miter;stroke-opacity:1\"\n         transform=\"translate(5010.6777,942.8175)\" /></g></g><path\n     d=\"M 19657.6 32703.7 C 19692.2 32408.2 19726.9 32124.8 19761.6 32036.9 C 19796.2 31949 19830.9 32064.5 19865.6 32307.7 C 19900.2 32551 19934.9 32903 19969.6 33135.3 C 20004.2 33367.7 20038.9 33461.2 20073.6 33356 C 20108.2 33250.7 20142.9 32954.3 20177.6 32659.4 C 20212.2 32364.5 20246.9 32094.9 20281.6 32025.1 C 20316.2 31955.3 20350.9 32091.6 20385.6 32345 C 20420.2 32598.4 20454.9 32949 20489.6 33169.3 C 20524.3 33389.6 20558.9 33461.4 20593.6 33338.9 C 20628.3 33216.3 20662.9 32908.4 20697.6 32615.3 C 20732.3 32322.2 20766.9 32067.5 20801.6 32016 C 20836.3 31964.5 20870.9 32121.2 20905.6 32383.7 C 20940.3 32646.2 20974.9 32994 21009.6 33201.3 C 21044.3 33408.7 21078.9 33458.5 21113.6 33319.2 C 21148.3 33179.8 21182.9 32861.7 21217.6 32571.5 C 21252.3 32281.4 21286.9 32042.7 21321.6 32009.7 C 21356.3 31976.8 21390.9 32153.1 21425.6 32423.7 C 21460.3 32694.3 21494.9 33037.8 21529.6 33231.4 C 21564.3 33425 21598.9 33452.6 21633.6 33297 C 21668.3 33141.4 21702.9 32814.3 21737.6 32528.3 C 21772.3 32242.3 21806.9 32020.5 21841.6 32006.2 C 21876.3 31992 21910.9 32187.3 21945.6 32464.9 C 21980.3 32742.4 22014.9 33080.3 22049.6 33259.3 C 22084.3 33438.4 22119 33443.7 22153.6 33272.5 C 22188.3 33101.3 22223 32766.6 22257.6 32485.8 C 22292.3 32205.1 22327 32001 22361.6 32005.5 C 22396.3 32010 22431 32223.5 22465.6 32507 C 22500.3 32790.4 22535 33121.2 22569.6 33285 C 22604.3 33448.9 22639 33431.8 22673.6 33245.6 C 22708.3 33059.5 22743 32718.5 22777.6 32444.2 C 22812.3 32169.8 22847 31984.4 22881.6 32007.6 C 22916.3 32030.8 22951 32261.7 22985.6 32549.9 C 23020.3 32838 23055 33160.5 23089.6 33308.4 C 23124.3 33456.3 23159 33417 23193.6 33216.6 C 23228.3 33016.3 23263 32670.4 23297.6 32403.6 C 23332.3 32136.7 23367 31970.7 23401.6 32012.5 C 23436.3 32054.4 23471 32301.7 23505.6 32593.4 C 23540.3 32885.1 23575 33198 23609.6 33329.3 C 23644.3 33460.7 23679 33399.2 23713.6 33185.5 C 23748.3 32971.9 23783 32622.5 23817.7 32364.2 C 23852.3 32105.9 23887 31959.9 23921.7 32020.2 C 23956.3 32080.5 23991 32343.2 24025.7 32637.3 C 24060.3 32931.4 24095 33233.4 24129.7 33347.7 C 24164.3 33462.1 24199 33378.7 24233.7 33152.5 C 24268.3 32926.3 24303 32574.8 24337.7 32326.2 C 24372.3 32077.5 24407 31952.1 24441.7 32030.7 C 24476.3 32109.2 24511 32386.2 24545.7 32681.5 C 24580.3 32976.8 24615 33266.7 24649.7 33363.6 C 24684.3 33460.4 24719 33355.5 24753.7 33117.7 C 24788.3 32879.9 24823 32527.7 24857.7 32289.7 C 24892.3 32051.7 24927 31947.4 24961.7 32043.8 C 24996.3 32140.3 25031 32430.5 25065.7 32725.8 C 25100.3 33021.1 25135 33297.8 25169.7 33376.7 C 25204.3 33455.6 25239 33329.6 25273.7 33081.2 C 25308.3 32832.8 25343 32481.3 25377.7 32254.9 C 25412.3 32028.4 25447 31945.7 25481.7 32059.6 C 25516.4 32173.6 25551 32475.9 25585.7 32770.1 C 25620.4 33064.2 25655 33326.5 25689.7 33387.2 C 25724.4 33447.8 25759 33301.3 25793.7 33043.2 C 25828.4 32785.1 25863 32435.8 25897.7 32221.8 C 25932.4 32007.9 25967 31947 26001.7 32078 C 26036.4 32209.1 26071 32522.3 26105.7 32814 C 26140.4 33105.8 26175 33352.6 26209.7 33394.8 C 26244.4 33437.1 26279 33270.5 26313.7 33003.8 C 26348.4 32737.1 26383 32391.3 26417.7 32190.7 C 26452.4 31990.1 26487 31951.4 26521.7 32099 C 26556.4 32246.5 26591 32569.3 26625.7 32857.5 C 26660.4 33145.8 26695 33376.2 26729.7 33399.8 C 26764.4 33423.4 26799 33237.4 26833.7 32963.2 C 26868.4 32689 26903 32348.2 26937.7 32161.7 C 26972.4 31975.3 27007 31958.8 27041.7 32122.3 C 27076.4 32285.8 27111 32616.9 27145.7 32900.4 C 27180.4 33183.9 27215.1 33397 27249.7 33401.9 C 27284.4 33406.7 27319.1 33202.2 27353.7 32921.6 C 27388.4 32640.9 27423.1 32306.4 27457.7 32134.9 C 27492.4 31963.4 27527.1 31969.3 27561.7 32148 C 27596.4 32326.8 27631.1 32664.8 27665.7 32942.5 C 27700.4 33220.2 27735.1 33415 27769.7 33401.2 C 27804.4 33387.3 27839.1 33165 27873.7 32879.1 C 27908.4 32593.1 27943.1 32266.3 27977.7 32110.4 C 28012.4 31954.4 28047.1 31982.6 28081.7 32176 C 28116.4 32369.3 28151.1 32712.9 28185.7 32983.6 C 28220.4 33254.4 28255.1 33430.2 28289.7 33397.7 C 28324.4 33365.1 28359.1 33125.9 28393.7 32835.8 C 28428.4 32545.8 28463.1 32227.9 28497.7 32088.2 C 28532.4 31948.5 28567.1 31998.9 28601.7 32206 C 28636.4 32413.2 28671.1 32761 28705.7 33023.7 C 28740.4 33286.3 28775.1 33442.5 28809.8 33391.3 C 28844.4 33340.2 28879.1 33085.1 28913.8 32792.1 C 28948.4 32499 28983.1 32191.4 29017.8 32068.5 C 29052.4 31945.6 29087.1 32018 29121.8 32238.1 C 29156.4 32458.2 29191.1 32808.8 29225.8 33062.4 C 29260.4 33316 29295.1 33451.7 29329.8 33382.3 C 29364.4 33312.8 29399.1 33042.8 29433.8 32748 C 29468.4 32453.1 29503.1 32157 29537.8 32051.4 C 29572.4 31945.8 29607.1 32039.9 29641.8 32272 C 29676.4 32504.2 29711.1 32856.2 29745.8 33099.6 C 29780.4 33343.1 29815.1 33458 29849.8 33370.5 C 29884.4 33282.9 29919.1 32999.1 29953.8 32703.7\"\n     id=\"path3\"\n     style=\"fill:none;stroke:#00ff00;stroke-width:100;paint-order:fill markers stroke;stroke-dasharray:none\"\n     title=\"t sin(20*t)\" /></svg>"
  w66 = string[] ["<path", "<rect", "<circle", "<g"]
  w95 = string[] ["<path", "<rect", "<circle", "<g"]
  w142 = path "C:/Users/Albro/Documents/GitHub/AFM-Lithography/test files/Overlay Testing.svg" ("Path")
  # "Split up the string at end of specified object"
  # "This will find and dynamically edit the svg so it can be updated properly"
  # "For this to work:\nI should have a unique name for the file that is possible to find layer and update later as well\nI need to have a robust way of determining the background and the overlay images, and identifying them from all of the other stuff in the file\nI will need to be able to search for all of the images, and either\nA) Insert a new overlay file into the SVG\nB) Replace an existing overlay file in the SVG\nFor scenario A) \nThis will involve:\ngenerating XML, \na unique ID for the image object, \nsetting up the URI for the image relative to the SVG file location\nCalculating the offsets\nCalculating the width and height"
  # "What needs to be done now:\nFind all IDs in the file\nGenerate a unique ID\nFind relative difference in position of two images"
  n1 = Match Pattern(string=w8, regular expression=">") -> (offset past match=→"offset past match 5":i32)  [unwired: 1 in, 3 out]
  n2 = Match Pattern(string=w8, regular expression="</") -> (offset past match=→"offset past match 4":i32)  [unwired: 1 in, 3 out]
  n3 = Match Pattern(string=w8, regular expression="/>") -> (offset past match=→"offset past match 2":i32)  [unwired: 1 in, 3 out]
  n4 = Match Pattern(string=w8, regular expression="<!--") -> (after substring=w2:string, offset past match=→"offset past match 3":i32)  [unwired: 1 in, 2 out]
  n5 = call "Write RawXML.vi"("RawXML"=w37, "ParseSVG.lvclass"=refnum<class "ParseSVG.lvclass"> refnum ("ParseXML in")) -> ("ParseSVG.lvclass 2"=w50:refnum<class "ParseSVG.lvclass">)  [unwired: 8 in, 1 out]
  n6 = while {
    shift-right: [w154] -> _
    shift-left: w37 -> [w154]
    shift-right: [w152] -> _
    shift-left: 0 -> [w159]
    tunnel: [w157] -> w35 mode=indexing if=w147
    tunnel: "<g" -> [w149]
    tunnel: [w150] -> w40 mode=indexing if=w147
    tunnel: [w152] -> w16 mode=indexing if=w147
    shift-right: [w150] -> _
    shift-left: 0 ("offset past match") -> [w151]
    tunnel: [w148] -> _ mode=indexing if=w147
    stop <- w156 stop-if-true
    # "removed increments here"
    # "Find all of the starts of the groups"
    # "find all of the ends of the groups"
    n7 = Match Pattern(string=w154, regular expression=w149, offset (0)=w159) -> (offset past match=w148:i32)  [unwired: 3 out]
    n8 = String Subset(string=w154, offset (0)=w148) -> (substring=w160:string)  [unwired: 1 in]
    n9 = Less Than 0?(x=w148) -> (x < 0?=w156:bool)
    n10 = Match Pattern(string=w160, regular expression=">") -> (before substring=w157:string, offset past match=w155:i32)  [unwired: 1 in, 2 out]
    n11 = Add(x=w155, y=w148) -> (x+y=w152:i32)
    n12 = Match Pattern(string=w154, regular expression="</g>", offset (0)=w151) -> (offset past match=w150:i32)  [unwired: 3 out]
    n13 = Not(x=w156) -> (.not. x?=w147:bool)
  }
  "Array" <- w16
  n14 = while {
    shift-right: [w165] -> _
    shift-left: w37 -> [w165]
    shift-right: [w164] -> _
    shift-left: 0 -> [w170]
    tunnel: [w168] -> w31 mode=indexing if=w161
    tunnel: "<path" -> [w163]
    tunnel: [w164] -> w33 mode=indexing if=w161
    tunnel: [w162] -> w32 mode=indexing if=w161
    stop <- w167 stop-if-true
    # "removed increments here"
    # "Find all of the starts of the groups"
    # "find all of the ends of the groups"
    n15 = Match Pattern(string=w165, regular expression=w163, offset (0)=w170) -> (offset past match=w162:i32)  [unwired: 3 out]
    n16 = String Subset(string=w165, offset (0)=w162) -> (substring=w171:string)  [unwired: 1 in]
    n17 = Less Than 0?(x=w162) -> (x < 0?=w167:bool)
    n18 = Match Pattern(string=w171, regular expression="/>") -> (before substring=w168:string, offset past match=w166:i32)  [unwired: 1 in, 2 out]
    n19 = Add(x=w166, y=w162) -> (x+y=w164:i32)
    n20 = Not(x=w167) -> (.not. x?=w161:bool)
  }
  "Array 2" <- w33
  "Array 3" <- w32
  n21 = Concatenate Strings("<" ("regular expression"), "path" ("string")) -> (w52:string)
  n22 = call-dynamic "Write Path.vi"("Path"=w142, "ParseSVG in"=refnum<class "ParseSVG.lvclass"> refnum) -> ("error out"=w138:errorcluster, "ParseSVG out"=w146:refnum<class "ParseSVG.lvclass">)  [unwired: 8 in]
  n23 = Open/Create/Replace File(file path (use dialog)=w142) -> (refnum out=w143:refnum<file>, error out=w133:errorcluster)  [unwired: 5 in, 1 out]
  n24 = Match Pattern(string=w2, regular expression="-->") -> (after substring=→"after substring":string)  [unwired: 1 in, 3 out]
  n25 = while {
    shift-right: [w182] -> _
    shift-left: w37 -> [w182]
    shift-right: [w175] -> _
    shift-left: 0 -> [w180]
    tunnel: [w178] -> _ mode=indexing if=w172
    tunnel: [w175] -> w48 mode=indexing if=w172
    tunnel: w52 -> [w174]
    tunnel: [w173] -> w49 mode=indexing if=w172
    stop <- w177 stop-if-true
    # "removed an increment here"
    n26 = Match Pattern(string=w182, regular expression=w174, offset (0)=w180) -> (offset past match=w173:i32)  [unwired: 3 out]
    n27 = String Subset(string=w182, offset (0)=w173) -> (substring=w181:string)  [unwired: 1 in]
    n28 = Less Than 0?(x=w173) -> (x < 0?=w177:bool)
    n29 = Match Pattern(string=w181, regular expression="/>") -> (before substring=w178:string, offset past match=w176:i32)  [unwired: 1 in, 2 out]
    n30 = Add(x=w176, y=w173) -> (x+y=w175:i32)
    n31 = Not(x=w177) -> (.not. x?=w172:bool)
  }
  "path start" <- w49
  "Path End" <- w48
  n32 = Read from Text File(file (use dialog)=w143, error in=w133) -> (refnum out=w139:refnum<file>, text=w141:string, error out=w140:errorcluster)  [unwired: 2 in, 1 out]
  n33 = call "Get Groups.vi"("ParseSVG in"=w50) -> ("ParseSVG out"=w47:refnum<class "ParseSVG.lvclass">)  [unwired: 9 in, 1 out]
  n34 = call "Write RawXML.vi"("error in (no error)"=w138, "RawXML"=w141, "ParseSVG.lvclass"=w146) -> ("error out"=w144:errorcluster, "ParseSVG.lvclass 2"=w88:refnum<class "ParseSVG.lvclass">)  [unwired: 7 in]
  n35 = disable-structure shown="Disabled" {
    disable-tunnel: [w185 _] -> w56
    frame Disabled {
      n36 = call "Insert Image Blank File Size Dialogue.vi"("Message to User"="There was no ", "Scan Size (um)"=30.0) -> ("Error Out"=w185:errorcluster)  [unwired: 7 in, 2 out]
    }
    frame Enabled {
    }
  }
  n37 = Close File(refnum=w139, error in=w140) -> (error out=w135:errorcluster)  [unwired: 1 out]
  n38 = call-dynamic "Read Groups.vi"("ParseSVG in"=w47) -> ("Groups"=→"Groups":T1)  [unwired: 8 in, 2 out]
  n39 = call "Get Images.vi"("error in (no error)"=w144, "ParseSVG in"=w88) -> ("ParseSVG out"=w134:refnum<class "ParseSVG.lvclass">)  [unwired: 8 in, 1 out]
  n40 = Match Pattern(string=w37, regular expression="</g>") -> (offset past match=→"offset past match":i32)  [unwired: 1 in, 3 out]
  n41 = call "Read RawXML.vi"("error in (no error)"=w56, "ParseXML in"=refnum<class "ParseSVG.lvclass"> refnum) -> ("RawXML"=w70:string, "ParseXML out"=w104:refnum<class "ParseSVG.lvclass">)  [unwired: 7 in, 1 out]
  n42 = call "Find SVG Object.vi"("Ending Delimiter"="\"", "Beginning Delimiter"="id=\"", "XML String"=w70) -> ("Found Values"=w74:string[])  [unwired: 6 in, 2 out]
  n43 = Reverse 1D Array(array=w40) -> (reversed array=w36:i32[])
  n44 = while {
    shift-right: [w189] -> _
    shift-left: w74 -> [w189]
    tunnel: "image " -> [w191]
    tunnel: [w188] -> w72
    i -> [w192]
    stop <- w187 stop-if-true
    n45 = Number To Decimal String(number=w192) -> (decimal integer string=w186:string)  [unwired: 1 in]
    n46 = Concatenate Strings(w191, w186) -> (w188:string)
    n47 = Search 1D Array(1D array=w189, element=w188) -> (index of element=w190:i32)  [unwired: 1 in]
    n48 = Less Than 0?(x=w190) -> (x < 0?=w187:bool)
  }
  n49 = call "Read Images.vi"("error in (no error)"=w135, "ParseSVG in"=w134) -> ("error out"=w137:errorcluster, "Images"=w131:T5[], "ParseSVG out"=w136:refnum<class "ParseSVG.lvclass">)  [unwired: 7 in]
  n50 = call "Find SVG Object.vi"("Ending Delimiter"="\"", "Beginning Delimiter"="id=\"", "XML String"="RawXML") -> ("Found Values"=w92:string[])  [unwired: 6 in, 2 out]
  n51 = for {
    tunnel: w34 -> [w194]
    tunnel: w36 -> [w197] mode=indexing
    tunnel: w16 -> [w196] mode=indexing
    tunnel: w35 -> [w195] mode=indexing
    tunnel: [w193] -> w30 mode=indexing
    n52 = Bundle By Name(cluster=w194, "End"=w197, "attributes"=w195, "Start"=w196) -> (w193:T4)
  }
  n53 = for {
    tunnel: w34 -> [w202]
    tunnel: w33 -> [w201] mode=indexing
    tunnel: w32 -> [w200] mode=indexing
    tunnel: w31 -> [w199] mode=indexing
    tunnel: [w198] -> w29 mode=indexing
    n54 = Bundle By Name(cluster=w202, "Start"=w200, "attributes"=w199, "End"=w201) -> (w198:T4)
  }
  n55 = while {
    shift-right: [w205] -> _
    shift-left: w92 -> [w205]
    tunnel: "image " -> [w207]
    tunnel: [w204] -> w87
    i -> [w209]
    stop <- w203 stop-if-true
    n56 = Number To Decimal String(number=w209) -> (decimal integer string=w208:string)  [unwired: 1 in]
    n57 = Concatenate Strings(w207, w208) -> (w204:string)
    n58 = Search 1D Array(1D array=w205, element=w204) -> (index of element=w206:i32)  [unwired: 1 in]
    n59 = Less Than 0?(x=w206) -> (x < 0?=w203:bool)
  }
  n60 = call <vilib>:"Define Criteria.vi"("Criteria"=Criteria."Globally-Unique Name") -> ("UniquenessCriteria out"=w17:refnum<class "UniquenessCriteria.lvclass">)  [unwired: 10 in]
  n61 = call <vilib>:"Default Registry Configuration.vi"() -> ("Registry Configuration"=w19:T6)  [unwired: 11 in]
  n62 = Bundle By Name(cluster=w19, "UniquenessCriteria"=w17) -> (w18:T6)
  n63 = call-dynamic "Read Path.vi"("ParseSVG in"=w104) -> ("Path"=w83:path, "ParseSVG out"=w65:refnum<class "ParseSVG.lvclass">)  [unwired: 8 in, 1 out]
  n64 = call "Get Background Image Relative Path.vi"("Inkscape Path"=path "C:/Users/Albro/Documents/GitHub/AFM-Lithography/test files/Overlay Testing/Test No Image/TestNoIMage.svg") -> ("Relative Path to Background"=w103:path)  [unwired: 2 in]
  n65 = call <vilib>:"Create Registry.vi"("Registry Configuration"=w18) -> ("Registry"=w28:refnum<data-value>)  [unwired: 9 in, 1 out]
  n66 = Path To String(path=w103) -> (string=w101:string)
  n67 = call "Get Background Image Relative Path.vi"("Inkscape Path"=w83) -> ("Relative Path to Background"=w84:path)  [unwired: 2 in]
  n68 = call <vilib>:"Register Item.vi"("Registry in"=w28) -> ("Registry"=w27:refnum<data-value>)  [unwired: 8 in, 2 out]
  n69 = Path To String(path=w84) -> (string=w82:string)
  n70 = for {
    tunnel: w30 -> [w217] mode=indexing
    shift-right: [w211] -> w15
    shift-left: w27 -> [w214]
    shift-right: [w210] -> w13
    shift-left: w29 -> [w218]
    n71 = Concatenate Strings("group" ("string")) -> (w215:string)
    n72 = call <vilib>:"Register Item.vi"("New Object Name"=w215, "Registry in"=w214) -> ("New Node"=w212:refnum<class "UniqueName.lvclass">, "Registry"=w213:refnum<data-value>)  [unwired: 7 in, 1 out]
    n73 = for {
      tunnel: w218 -> [w221] mode=indexing
      tunnel: w217 -> [w227]
      tunnel: w212 -> [w225]
      shift-right: [w224] -> w211
      shift-left: w213 -> [w226]
      tunnel: [w221] -> w210 mode=indexing if=w220
      n74 = Unbundle By Name(w221) -> ("Start"=w228:i32)
      n75 = Unbundle By Name(w227) -> ("Start"=w222:i32, "End"=w223:i32)
      n76 = In Range and Coerce(upper limit=w223, x=w228, lower limit=w222) -> (In Range?=w219:bool)  [unwired: 1 out]
      n77 = case shown="True" w219 {
        tunnel: w226 -> [w229 w233]
        tunnel: w225 -> [_ w232]
        tunnel: [w229 w230] -> w224
        frame False {
        }
        frame True {
          n78 = call <vilib>:"Register Item.vi"("Owner"=w232, "New Object Name"="path" ("string"), "Registry in"=w233) -> ("Registry"=w230:refnum<data-value>)  [unwired: 6 in, 2 out]
        }
      }
      n79 = Not(x=w219) -> (.not. x?=w220:bool)
    }
  }
  n80 = Array Size(array=w95) -> (size(s)=w110:i32)
  n81 = Bundle By Name(cluster=T5 {"x"="", "y"="", "width"="", "height"="", "xlink:href"="", "id"="", "transform"=""} ("image"), "xlink:href"=w82, "x"="0", "y"="0", "width"="30000", "height"="30000", "id"=w72) -> (w64:T5)
  n82 = for {
    shift-right: [w261] -> w117
    shift-left: w137 -> [w253]
    tunnel: w131 -> [w242] mode=indexing
    shift-right: [w248] -> w118
    shift-left: w136 -> [w254]
    tunnel: [w262] -> w130 mode=indexing
    tunnel: [w257] -> w129 mode=indexing
    tunnel: [w239] -> w120 mode=indexing
    tunnel: [w234] -> w116 mode=indexing
    i -> [w256]
    n83 = call-dynamic "Read Path.vi"("error in (no error)"=w253, "ParseSVG in"=w254) -> ("error out"=w252:errorcluster, "Path"=w250:path, "ParseSVG out"=w249:refnum<class "ParseSVG.lvclass">)  [unwired: 7 in]
    n84 = Unbundle By Name(w242) -> ("x"=w266:string, "y"=w265:string, "width"=w264:string, "height"=w263:string, "id"=w247:string, "xlink:href"=w251:string)
    n85 = call "Check Embedded.vi"("SVG Path"=w250, "error in (no error)"=w252, "URI"=w251) -> ("error out"=w255:errorcluster, "Embedded"=w234:bool, "Path Out"=w243:string)  [unwired: 6 in]
    n86 = Bundle By Name(cluster=T7 {"X"="", "Y"="", "Width"="", "Height"="", "File Path"="", "ID"="", "transform"=""} ("Info"), "X"=w266, "Y"=w265, "Width"=w264, "Height"=w263, "ID"=w247, "File Path"=w243) -> (w259:T7)
    n87 = call "Initialize.vi"("error in (no error)"=w255, "Info"=w259, "Image in"=refnum<class "SVGImage.lvclass"> refnum) -> ("error out"=w238:errorcluster, "Image out"=w241:refnum<class "SVGImage.lvclass">)  [unwired: 7 in]
    n88 = call "Read RawXML.vi"("error in (no error)"=w238, "ParseXML in"=w249) -> ("error out"=w237:errorcluster, "RawXML"=w245:string, "ParseXML out"=w246:refnum<class "ParseSVG.lvclass">)  [unwired: 7 in]
    n89 = case shown="True" w234 {
      tunnel: [w269 w278] -> w236
      tunnel: w237 -> [w269 w277]
      tunnel: w245 -> [w268 w276]
      tunnel: [w268 w275] -> w244
      tunnel: w243 -> [_ w274]
      tunnel: w242 -> [w267 w271]
      tunnel: w241 -> [w270 w273]
      tunnel: [w270 w272] -> w240
      tunnel: [w267 w271] -> w239
      frame False {
      }
      frame True {
        n90 = call "Replace Embedded SVG.vi"("image"=w271, "error in"=w277, "xlink:href"=w274, "XML In"=w276, "SVGImage in"=w273) -> ("error out"=w278:errorcluster, "Edited XML Out"=w275:string, "SVGImage out"=w272:refnum<class "SVGImage.lvclass">)  [unwired: 3 in, 1 out]
      }
    }
    n91 = call "Write RawXML.vi"("error in (no error)"=w236, "RawXML"=w244, "ParseSVG.lvclass"=w246) -> ("error out"=w235:errorcluster, "ParseSVG.lvclass 2"=w248:refnum<class "ParseSVG.lvclass">)  [unwired: 7 in]
    n92 = call "IsTempBackground.vi"("SVG Path"=w250, "error in"=w235, "Order (back to front)"=w256, "SVGImage in"=w240) -> ("error out"=w261:errorcluster, "Backgroundic Qualities"=w257:T8, "SVGImage out"=w262:refnum<class "SVGImage.lvclass">)  [unwired: 5 in]
  }
  n93 = call "Generate SVG Attribute Object.vi"("Named Cluster of Data"=w64) -> ("SVG Attribute Object"=w59:string)  [unwired: 9 in, 1 out]
  n94 = for {
    N: w110 -> [_]
    tunnel: "RawXML" -> [w282]
    tunnel: w95 -> [w281] mode=indexing
    tunnel: string[] ["/>", "/>", "/>", "</g>"] -> [w280] mode=indexing
    tunnel: [w279] -> w108 mode=concatenating
    n95 = call "Find SVG Object.vi"("Ending Delimiter"=w280, "Beginning Delimiter"=w281, "XML String"=w282) -> ("Beginning Indices"=w279:i32[])  [unwired: 6 in, 2 out]
  }
  n96 = call "Read RawXML.vi"("ParseXML in"=w65) -> ("RawXML"=w62:string, "ParseXML out"=w58:refnum<class "ParseSVG.lvclass">)  [unwired: 8 in, 1 out]
  n97 = Bundle By Name(cluster=T5 {"x"="", "y"="", "width"="", "height"="", "xlink:href"="", "id"="", "transform"=""} ("image"), "x"="0", "y"="0", "xlink:href"=w101, "width"="30000", "height"="30000" ("transform"), "id"=w87) -> (w99:T5)
  n98 = Array Max & Min(array=w108) -> (min value=w85:i32)  [unwired: 3 out]
  n99 = call "Generate SVG Attribute Object.vi"("Named Cluster of Data"=w99) -> ("SVG Attribute Object"=w105:string)  [unwired: 9 in, 1 out]
  n100 = Array Size(array=w66) -> (size(s)=w69:i32)
  n101 = for {
    N: w69 -> [_]
    tunnel: w62 -> [w286]
    tunnel: w66 -> [w285] mode=indexing
    tunnel: string[] ["/>", "/>", "/>", "</g>"] -> [w284] mode=indexing
    tunnel: [w283] -> w67 mode=concatenating
    n102 = call "Find SVG Object.vi"("Ending Delimiter"=w284, "Beginning Delimiter"=w285, "XML String"=w286) -> ("Beginning Indices"=w283:i32[])  [unwired: 6 in, 2 out]
  }
  n103 = for {
    shift-right: [w288] -> w14
    shift-left: w15 -> [w289]
    tunnel: w13 -> [_] mode=indexing
    n104 = call <vilib>:"Register Item.vi"("New Object Name"="path", "Registry in"=w289) -> ("Registry"=w288:refnum<data-value>)  [unwired: 7 in, 2 out]
  }
  n105 = String Subset(string="RawXML", offset (0)=w85) -> (substring=w107:string)  [unwired: 1 in]
  n106 = String Subset(string="RawXML", length (rest)=w85) -> (substring=w106:string)  [unwired: 1 in]
  n107 = Array Max & Min(array=w67) -> (min value=w63:i32)  [unwired: 3 out]
  n108 = String Subset(string=w62, offset (0)=w63) -> (substring=w60:string)  [unwired: 1 in]
  n109 = String Subset(string=w62, length (rest)=w63) -> (substring=w61:string)  [unwired: 1 in]
  n110 = call <vilib>:"Query Registry.vi"("use Regex? (F)"=TRUE, "Search string"=".*", "Search Key (FQN)"=Key."Fully Qualified Name", "Registry in"=w14) -> ("Nodes"=w23:refnum<class "UniqueName.lvclass">[], "Registry"=w21:refnum<data-value>)  [unwired: 3 in, 3 out]
  n111 = Concatenate Strings(w106, w105, w107) -> (→"Edited in":string)
  n112 = Concatenate Strings(w61, w59, w60) -> (w57:string)
  n113 = for {
    tunnel: w23 -> [w291] mode=indexing
    tunnel: [w290] -> w22 mode=indexing
    n114 = call <vilib>:"Read Fully Qualified Name.vi"("UniqueName in"=w291) -> ("Fully Qualified Name"=w290:string)  [unwired: 9 in, 1 out]
  }
  "Array 4" <- w22
  n115 = call "Write RawXML.vi"("RawXML"=w57, "ParseSVG.lvclass"=w58) -> ()  [unwired: 8 in, 2 out]
  n116 = Or Array Elements(Boolean array=w116) -> (logical OR=w113:bool)
  n117 = call "Find Background Image.vi"("Backgroundic Qualities"=w129, "Images"=w130) -> ("Backgroundic Qualities"=w127:T8, "Background Image"=w128:refnum<class "SVGImage.lvclass">, "Index"=w122:i32)  [unwired: 7 in]
  n118 = Index Array(array=w120, index=w122) -> (element=w121:T5)
  n119 = Unbundle By Name(w127) -> ("Correct Name?"=w124:bool, "Surface Pic?"=w126:bool, "Correct Name?"=w125:bool)
  n120 = call <vilib>:"Destroy Registry.vi"("Registry in"=w21) -> ()  [unwired: 9 in, 2 out]
  n121 = Compound Arithmetic op=AND(w124, w126, w125) -> (w115:bool)
  n122 = Not(x=w115) -> (.not. x?=w114:bool)
  n123 = case shown="False" w115 {
    tunnel: w128 -> [w304 w312]
    tunnel: [w306 w313] -> w119
    tunnel: w118 -> [w310 w313]
    tunnel: [w305 w312] -> w123
    tunnel: w121 -> [w298 _]
    tunnel: w117 -> [w294 w311]
    tunnel: [w295 w311] -> w112
    frame False {
      # "Fix the data"
      n124 = call-dynamic "Read Path.vi"("error in (no error)"=w294, "ParseSVG in"=w310) -> ("error out"=w292:errorcluster, "Path"=w309:path, "ParseSVG out"=w303:refnum<class "ParseSVG.lvclass">)  [unwired: 7 in]
      n125 = call <vilib>:"Get File Extension.vi"("error in (no error)"=w292, "file"=w309) -> ("error out"=w293:errorcluster, "filename without extension"=w308:string)  [unwired: 5 in, 3 out]
      n126 = Concatenate Strings(w308, "_surfacepic.jpg" ("string")) -> (w299:string)
      n127 = call "Read RawXML.vi"("error in (no error)"=w293, "ParseXML in"=w303) -> ("error out"=w297:errorcluster, "RawXML"=w301:string, "ParseXML out"=w302:refnum<class "ParseSVG.lvclass">)  [unwired: 7 in]
      n128 = call "Replace Embedded SVG.vi"("image"=w298, "error in"=w297, "xlink:href"=w299, "XML In"=w301, "SVGImage in"=w304) -> ("error out"=w296:errorcluster, "Edited XML Out"=w300:string, "SVGImage out"=w305:refnum<class "SVGImage.lvclass">)  [unwired: 3 in, 1 out]
      n129 = call "Write RawXML.vi"("error in (no error)"=w296, "RawXML"=w300, "ParseSVG.lvclass"=w302) -> ("error out"=w295:errorcluster, "ParseSVG.lvclass 2"=w306:refnum<class "ParseSVG.lvclass">)  [unwired: 7 in]
    }
    frame True {
    }
  }
  "Background Image" <- w123
  n130 = Or(x=w114, y=w113) -> (x .or. y?=w111:bool)
  n131 = case shown="True" w111 {
    tunnel: w119 -> [_ w322]
    tunnel: w112 -> [w314 w316]
    tunnel: [w314 w318] -> w132
    frame False {
    }
    frame True {
      n132 = call-dynamic "Read Path.vi"("error in (no error)"=w316, "ParseSVG in"=w322) -> ("error out"=w317:errorcluster, "Path"=w320:path, "ParseSVG out"=w321:refnum<class "ParseSVG.lvclass">)  [unwired: 7 in]
      n133 = call "Read RawXML.vi"("error in (no error)"=w317, "ParseXML in"=w321) -> ("error out"=w315:errorcluster, "RawXML"=w324:string)  [unwired: 7 in, 1 out]
      n134 = Open/Create/Replace File(file path (use dialog)=w320, error in=w315) -> (refnum out=w323:refnum<file>, error out=w325:errorcluster)  [unwired: 4 in, 1 out]
      n135 = Write to Text File(file (use dialog)=w323, text=w324, error in=w325) -> (refnum out=w319:refnum<file>, error out=w326:errorcluster)  [unwired: 1 in, 1 out]
      n136 = Close File(refnum=w319, error in=w326) -> (error out=w318:errorcluster)  [unwired: 1 out]
    }
  }
  "error out" <- w132
